vi "Actor Core.vi"(8 "error in":errorcluster, 11 "Actor in":refnum<class "CAN Protocol Test.lvclass">) -> (0 "error out":errorcluster, 3 "Actor out":refnum<class "Actor.lvclass">)   [LabVIEW 2013, in "CAN Protocol Test.lvlib" / "CAN Protocol Test.lvclass"]
doc: "This is Actor Core.vi, the main message handling loop for Actors. An actor usually just sits in this loop and processes messages as they arrive. Any error returned by the message Do.vi call will stop the loop, with error code 43 as the cannonical signal to stop with no error sent to caller. Descendants may override that in Handle Error.vi."
uses:
  CAN Protocol Test.lvclass
  <vilib>/ActorFramework/Actor/Actor.lvclass
  CAN IO_class/CAN IO.lvclass
  _test class base/_test class base_Actor/_test class base.lvclass
  <vilib>/ActorFramework/Actor/Actor.lvclass/Actor.ctl
  <vilib>/ActorFramework/Message Enqueuer/Message Enqueuer.lvclass/Message Enqueuer.ctl
  _test class base/Messages/Send Status String to UI_Msg/Send Status String to UI_Msg.lvclass/Send Status String to UI_Msg.ctl
  <vilib>/ActorFramework/Message Enqueuer/Init from Existing Queue.vi
  <vilib>/ActorFramework/Message Enqueuer/Enqueue.vi
  <vilib>/ActorFramework/Message Priority Queue/Priority Enqueue.vi
  <vilib>/ActorFramework/Message Enqueuer/Message Enqueuer.lvclass
  _test class base/Messages/Send Status String to UI_Msg/Send Status String to UI_Msg.lvclass
  <vilib>/ActorFramework/Stop Msg/Stop Msg.lvclass
panel:
  out "Array":dbl[](array[numeric])
  in  "Type(5=DBL)":u8=255
  out "Numeric":i32
  in  "TLV Path(Tesla provided path)":path=path "C:/code/projects/Tesla/Tesla_testla/Ben submission/Data Files/test3.bin"
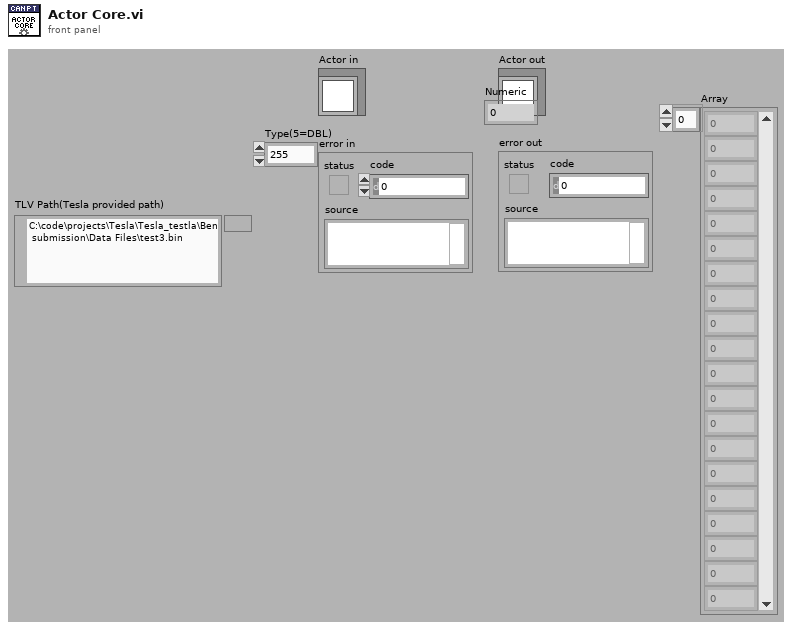
[diagram p1: front panel]
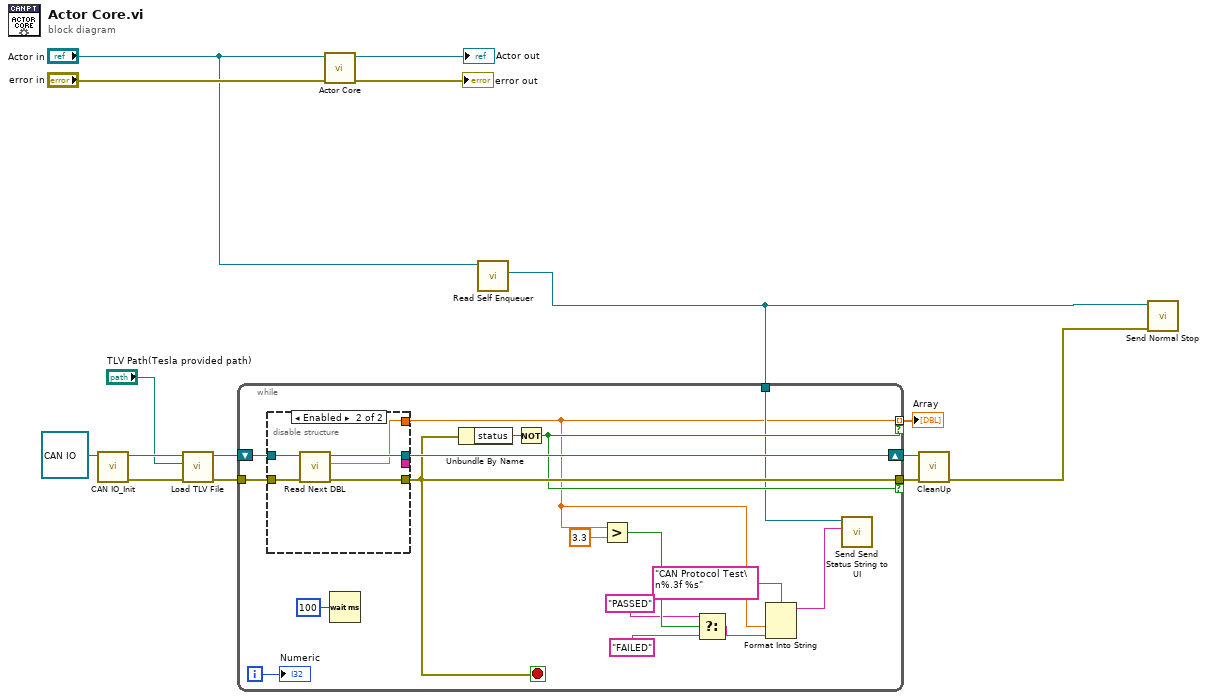
[diagram p0: block diagram]
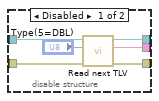
[diagram p2: hidden frame]
diagram:
  n1 = call "CAN IO_Init.vi"("object in"=refnum<class "CAN IO.lvclass"> refnum) -> ("error out"=w11:errorcluster, "object out"=w12:refnum<class "CAN IO.lvclass">)  [unwired: 9 in]
  n2 = call "Load TLV File.vi"("error in (no error)"=w11, "TLV Path"="TLV Path(Tesla provided path)", "object in"=w12) -> ("error out"=w9:errorcluster, "object out"=w10:refnum<class "CAN IO.lvclass">)  [unwired: 7 in]
  n3 = call-parent "Actor Core.vi"("error in"="error in", "Actor in"="Actor in") -> ("error out"=→"error out":errorcluster, "Actor out"=→"Actor out":refnum<class "Actor.lvclass">)  [unwired: 8 in]
  n4 = call <vilib>:"Read Self Enqueuer.vi"("Actor"="Actor in") -> ("Self Enqueuer"=w2:refnum<class "Message Enqueuer.lvclass">)  [unwired: 10 in]
  n5 = while {
    tunnel: w9 -> [w31]
    tunnel: [w29] -> w5 if=w26
    shift-right: [w30] -> w6
    shift-left: w10 -> [w32]
    tunnel: [w18] -> w4 mode=indexing if=w26
    tunnel: w2 -> [w24]
    i -> [w27]
    stop <- w29 stop-if-true
    n6 = disable-structure shown="Enabled" {
      disable-tunnel: w32 -> [w38 w43]
      disable-tunnel: w31 -> [w37 w42]
      disable-tunnel: [w36 w41] -> w30
      disable-tunnel: [w35 w39] -> w29
      disable-tunnel: [w34 _] -> _
      disable-tunnel: [_ w40] -> w18
      frame Disabled {
        n7 = call-dynamic "Read next TLV.vi"("error in (no error)"=w37, "Type(255=next available)"="Type(5=DBL)", "object in"=w38) -> ("error out"=w35:errorcluster, "TLV Payload"=w34:string, "object out"=w36:refnum<class "CAN IO.lvclass">)  [unwired: 6 in]
      }
      frame Enabled {
        n8 = call "Read Next DBL.vi"("error in (no error)"=w42, "object in"=w43) -> ("error out"=w39:errorcluster, "Value Read"=w40:dbl, "object out"=w41:refnum<class "CAN IO.lvclass">)  [unwired: 7 in]
      }
    }
    n9 = Wait (ms)(milliseconds to wait=u32 100) -> ()  [unwired: 1 out]
    n10 = Unbundle By Name(w29) -> ("status"=w28:bool)
    n11 = Not(x=w28) -> (.not. x?=w26:bool)
    n12 = Greater?(x=w18, y=3.3) -> (0:w21:bool)
    n13 = Select(t="PASSED" ("format string"), s=w21, f="FAILED" ("format string")) -> (s? t:f=w17:string)
    n14 = Format Into String(format string="CAN Protocol Test\n%.3f %s", w18, w17) -> (resulting string=w23:string)  [unwired: 2 in, 1 out]
    n15 = call "Send Send Status String to UI.vi"("Status String to Send"=w23, "Message Enqueuer"=w24) -> ()  [unwired: 8 in, 2 out]
    "Numeric" <- w27
  }
  "Array" <- w4
  n16 = call-dynamic "CleanUp.vi"("error in (no error)"=w5, "object in"=w6) -> ("error out"=w1:errorcluster)  [unwired: 8 in, 1 out]
  n17 = call <vilib>:"Send Normal Stop.vi"("error in (no error)"=w1, "Message Enqueuer"=w2) -> ()  [unwired: 9 in, 1 out]
